vi "SendCallbackMsg.vi"(8 "error in (no error)":errorcluster, 10 "UpstreamMsg":refnum<class "UpstreamMsgParent.lvclass">, 11 "DownStreamMsgHandler in":refnum<class "DownStreamMsgHandler.lvclass">) -> (0 "error out":errorcluster, 3 "DownStreamMsgHandler out":refnum<class "DownStreamMsgHandler.lvclass">)   [LabVIEW 2020, in "DownstreamMsgHandler.lvlib" / "DownStreamMsgHandler.lvclass"]
uses:
  DownStreamMsgHandler.lvclass
  C:/Program Files (x86)/National Instruments/LabVIEW 2020/vi.lib/ActorFramework/Actor/Actor.lvclass
  UpstreamMsg/UpstreamMsgParent/UpstreamMsgParent.lvclass
  <vilib>/ActorFramework/Actor/Actor.lvclass/Actor.ctl
  ServiceManager-Comms Messages/SendUpstreamMsg Msg/SendUpstreamMsg Msg.lvclass/SendUpstreamMsg Msg.ctl
  <vilib>/ActorFramework/Message Enqueuer/Message Enqueuer.lvclass/Message Enqueuer.ctl
  <vilib>/ActorFramework/Message Enqueuer/Enqueue.vi
  ServiceManager-Comms Messages/SendUpstreamMsg Msg/SendUpstreamMsg Msg.lvclass
  C:/Program Files (x86)/National Instruments/LabVIEW 2020/vi.lib/ActorFramework/Message/Message.lvclass
  <vilib>/ActorFramework/Message Priority Queue/Priority Enqueue.vi
  <vilib>/ActorFramework/Actor/Actor.lvclass
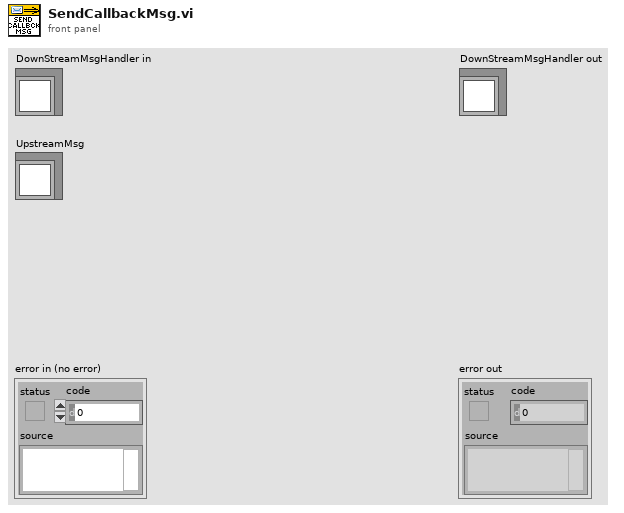
[diagram p1: front panel]
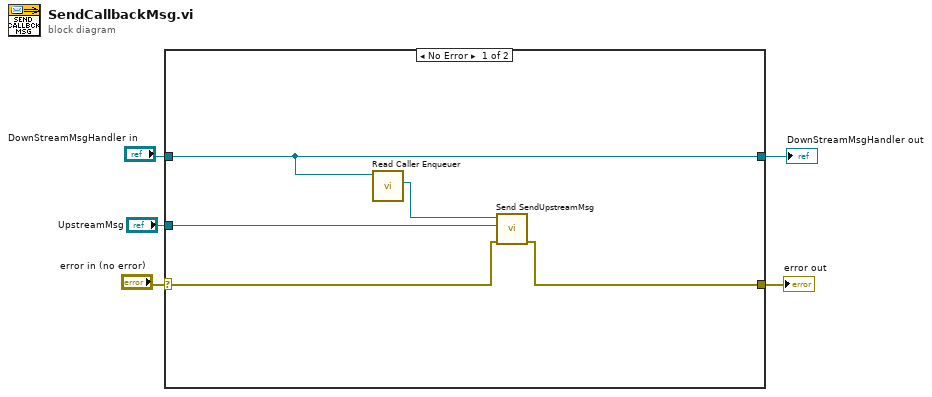
[diagram p0: block diagram]
diagram:
  n1 = case shown="No Error" "error in (no error)" {
    selector: "error in (no error)" -> [w10 w12]
    tunnel: [w9 w12] -> w4
    tunnel: [w8 w11] -> w2
    tunnel: "DownStreamMsgHandler in" -> [w8 w11]
    tunnel: "UpstreamMsg" -> [w6 _]
    frame No Error {
      n2 = call <vilib>:"Read Caller Enqueuer.vi"("Actor"=w8) -> ("Caller Enqueuer"=w7:refnum<class "Message Enqueuer.lvclass">)  [unwired: 10 in]
      n3 = call "Send SendUpstreamMsg.vi"("error in (no error)"=w10, "UpstreamMsg"=w6, "Message Enqueuer"=w7) -> ("error out"=w9:errorcluster)  [unwired: 7 in, 1 out]
    }
    frame Error {
    }
  }
  "error out" <- w4
  "DownStreamMsgHandler out" <- w2
